vi "GenSet_AE.vi"(7 "Enum":enum16{"READ", "WRITE"}(ring), 10 "General settings":T1 {"Mode Matrix" items=["Number", "Name"]}) -> (2 "General settings Out":T1 {"Mode Matrix" items=["Number", "Name"]})   [LabVIEW 2018]
uses:
  Controls/General Setting.ctl
  Controls/Buttons/Running Button.ctl
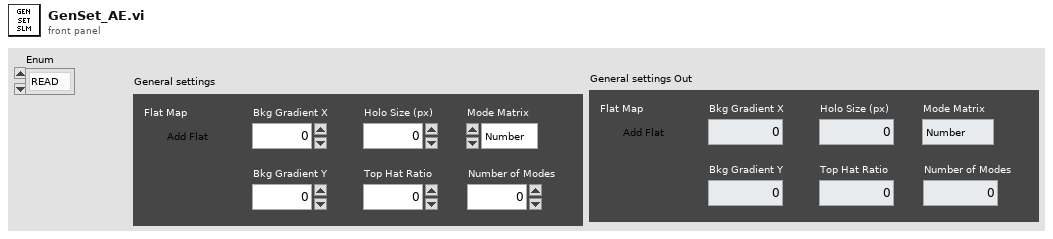
[diagram p1: front panel]
types:
  T1 = typedef "General Setting.ctl" = cluster{"Flat Map":T2, "Bkg Gradient X":dbl, "Bkg Gradient Y":dbl, "Holo Size (px)":i32, "Top Hat Ratio":dbl, "Number of Modes":i8, "Mode Matrix":u16}
  T2 = typedef "Running Button.ctl" = bool
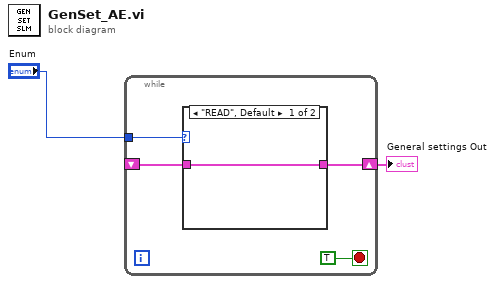
[diagram p0: block diagram]
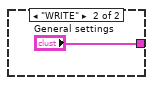
[diagram p2: hidden frame]
diagram:
  n1 = while {
    shift-right: [w5] -> w1
    shift-left: _ -> [w3]
    tunnel: "Enum" -> [w4]
    stop <- TRUE stop-if-true
    n2 = case shown="\"READ\", Default" w4 {
      tunnel: [w7 "General settings"] -> w5
      tunnel: w3 -> [w7 _]
      frame "READ", Default {
      }
      frame "WRITE" {
      }
    }
  }
  "General settings Out" <- w1
